vi "Entry.vi"(8 "error in (no error)":errorcluster, 11 "New State":refnum<class "Stopping Command.lvclass">) -> (0 "error out":errorcluster, 3 "State out":refnum<class "Stopping Command.lvclass">)   [LabVIEW 2014, in "Robot Actor Framework.lvlib" / "Command Processor Actor.lvlib" / "Stopping Command.lvclass"]
doc: "This is an abstract method. Override this method to define the behavior when you enter the state."
uses:
  Stopping Command.lvclass
  Command Processor Actor Class/Command Processor States.ctl
  <vilib>/ActorFramework/Message Enqueuer/Message Enqueuer.lvclass/Message Enqueuer.ctl
  <vilib>/ActorFramework/Message Enqueuer/Enqueue.vi
  <vilib>/ActorFramework/Message Priority Queue/Priority Enqueue.vi
  <vilib>/ActorFramework/Stop Msg/Stop Msg.lvclass
  Command Processor Actor Class/Command Processor Actor.lvclass
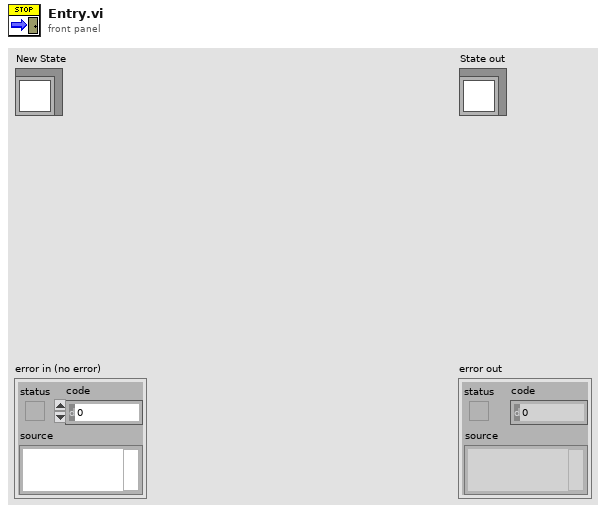
[diagram p1: front panel]
types:
  T1 = enum16{"Critical", "Error", "Warning", "Informational", "Debug"}
  T2 = typedef "Robot Actor Framework.lvlib/Command Processor Actor.lvlib/Command Processor Actor.lvclass/Command Processor States.ctl" = enum16{"Unknown", "No Command", "Running Command", "Starting Command", "Stopping Command", "Finishing Command"}
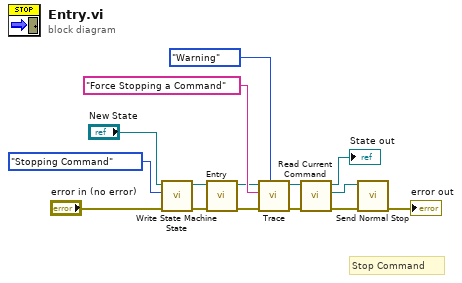
[diagram p0: block diagram]
diagram:
  # "Stop Command"
  n1 = call-dynamic "Write State Machine State.vi"("error in (no error)"="error in (no error)", "Command Processor State"=Command_Processor_States."Stopping Command", "Command Processor Actor in"="New State") -> ("error out"=w5:errorcluster, "Command Processor Actor out"=w6:refnum<class "Stopping Command.lvclass">)  [unwired: 7 in]
  n2 = call-parent "Entry.vi"("error in (no error)"=w5, "New State"=w6) -> ("error out"=w3:errorcluster, "State out"=w4:refnum<class "Stopping Command.lvclass">)  [unwired: 8 in]
  n3 = call-dynamic "Trace.vi"("Trace Level"=T1."Warning", "error in (no error)"=w3, "Command Processor Action"="Force Stopping a Command", "Command Processor Actor in"=w4) -> ("error out"=w9:errorcluster, "Command Processor Actor out"=w12:refnum<class "Stopping Command.lvclass">)  [unwired: 6 in]
  n4 = call-dynamic "Read Current Command.vi"("error in (no error)"=w9, "Command Processor in"=w12) -> ("error out"=w7:errorcluster, "Actor Framework:Message Enqueuer"=w8:refnum<class "Message Enqueuer.lvclass">, "Command Processor out"=→"State out":refnum<class "Stopping Command.lvclass">)  [unwired: 7 in]
  n5 = call <vilib>:"Send Normal Stop.vi"("error in (no error)"=w7, "Message Enqueuer"=w8) -> ("error out"=→"error out":errorcluster)  [unwired: 9 in]
